vi "SendTCPCommand.vi"(8 "error in (no error)":errorcluster, 9 "Command":string, 10 "Status":refnum<vi>, 11 "queue in":refnum<queue>) -> (0 "error out":errorcluster, 3 "queue out":refnum<queue>)   [LabVIEW 2016]
doc: "Sends command over TCP and updates status"
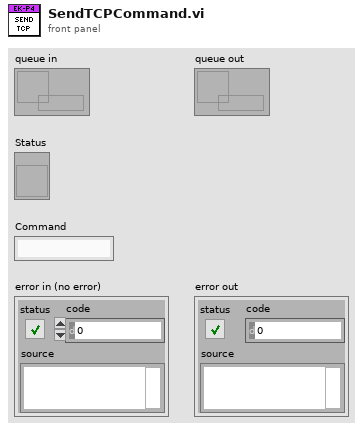
[diagram p1: front panel]
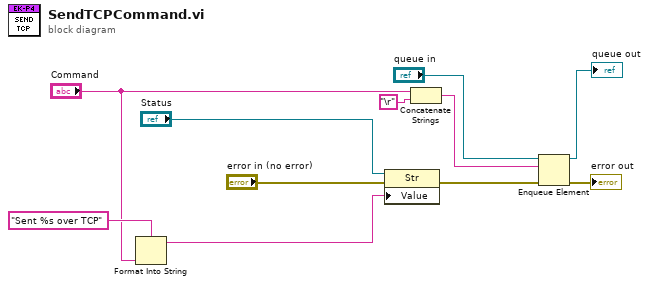
[diagram p0: block diagram]
diagram:
  n1 = Format Into String(format string="Sent %s over TCP", "Command") -> (resulting string=w5:string)  [unwired: 2 in, 1 out]
  n2 = property on="Property Node" class="Str"(reference="Status", error in="error in (no error)", "Value"=w5) -> (error out=w2:errorcluster)  [unwired: 1 out]
  n3 = Concatenate Strings("Command", "\r") -> (w11:string)
  n4 = Enqueue Element(queue="queue in", element=w11, error in (no error)=w2) -> (queue out=→"queue out":refnum<queue>, error out=→"error out":errorcluster)  [unwired: 1 in, 1 out]
